vi "GetRotation.vi"(7 "Game Ticks":u32, 8 "error in (no error)":errorcluster, 10 "Rotation Speed":sgl, 11 "Input in":refnum<class "Input.lvclass">) -> (0 "error out":errorcluster, 1 "Yaw":sgl, 2 "Pitch":sgl, 3 "Input out":refnum<class "Input.lvclass">)   [LabVIEW 2015, in "Input.lvclass"]
uses:
  Input.lvclass
  Input.lvclass/Input.ctl
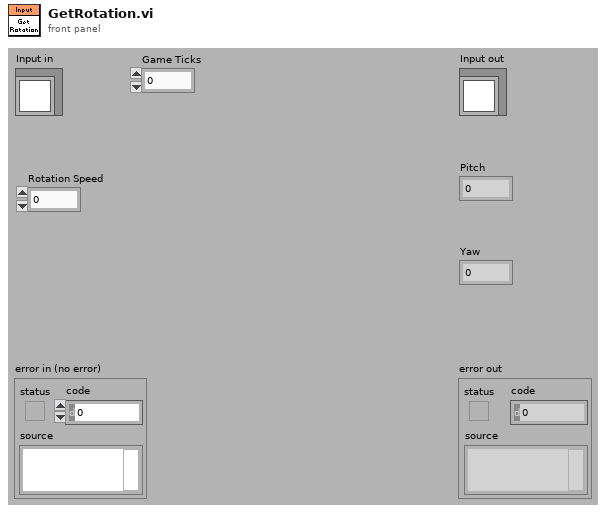
[diagram p1: front panel]
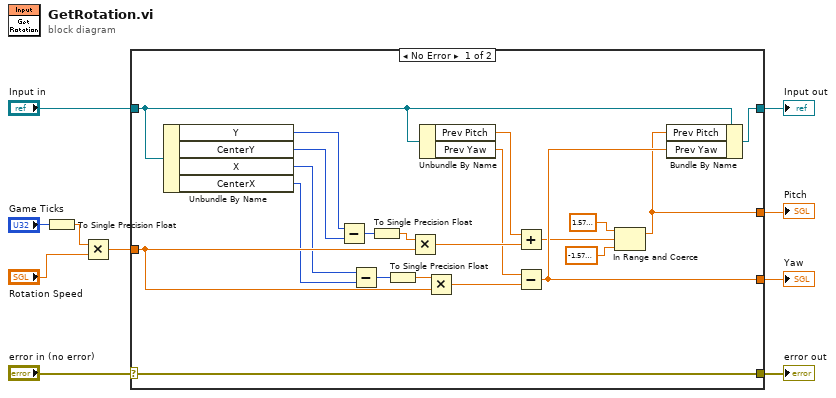
[diagram p0: block diagram]
diagram:
  n1 = To Single Precision Float(number="Game Ticks") -> (single precision float=w1:sgl)
  n2 = Multiply(x=w1, y="Rotation Speed") -> (x*y=w3:sgl)
  n3 = case shown="No Error" "error in (no error)" {
    selector: "error in (no error)" -> [w11 w33]
    tunnel: [w11 w33] -> w9
    tunnel: [w26 w32] -> w7
    tunnel: "Input in" -> [w16 w32]
    tunnel: w3 -> [w29 _]
    tunnel: [w23 _] -> w6
    tunnel: [w19 _] -> w5
    frame No Error {
      n4 = Unbundle By Name(w16) -> ("Y"=w13:i32, "CenterY"=w12:i32, "X"=w15:i32, "CenterX"=w14:i32)
      n5 = Subtract(x=w13, y=w12) -> (x-y=w17:i32)
      n6 = Subtract(x=w15, y=w14) -> (x-y=w18:i32)
      n7 = To Single Precision Float(number=w17) -> (single precision float=w30:sgl)
      n8 = To Single Precision Float(number=w18) -> (single precision float=w31:sgl)
      n9 = Multiply(x=w30, y=w29) -> (x*y=w27:sgl)
      n10 = Unbundle By Name(w16) -> ("Prev Pitch"=w28:sgl, "Prev Yaw"=w25:sgl)
      n11 = Multiply(x=w31, y=w29) -> (x*y=w24:sgl)
      n12 = Add(x=w28, y=w27) -> (x+y=w22:sgl)
      n13 = Subtract(x=w25, y=w24) -> (x-y=w23:sgl)
      n14 = In Range and Coerce(upper limit=sgl 1.57, x=w22, lower limit=sgl -1.57) -> (coerced(x)=w19:sgl)  [unwired: 1 out]
      n15 = Bundle By Name(cluster=w16, "Prev Pitch"=w19, "Prev Yaw"=w23) -> (w26:refnum<class "Input.lvclass">)
    }
    frame Error {
    }
  }
  "error out" <- w9
  "Input out" <- w7
  "Yaw" <- w6
  "Pitch" <- w5
